vi "getLimitsByName.vi"(8 "error in (no error)":errorcluster, 10 "device_name":string, 11 "deviceDataBase in":refnum<class "deviceDataBase.lvclass">) -> (0 "error out":errorcluster, 2 "Limits":T1(array[cluster]), 3 "deviceDataBase out":refnum<class "deviceDataBase.lvclass">)   [LabVIEW 2011, in "Tools.lvlib" / "DatabaseHelpers.lvlib" / "deviceDataBase.lvclass"]
uses:
  deviceDataBase.lvclass
  deviceDataBase.lvclass/deviceDataBase.ctl
  Database Objects/device/device.lvclass
  Database Objects/device/AnalogDevice/AnalogDevice.lvclass
  Database Objects/DeviceArray/DeviceArray.lvclass
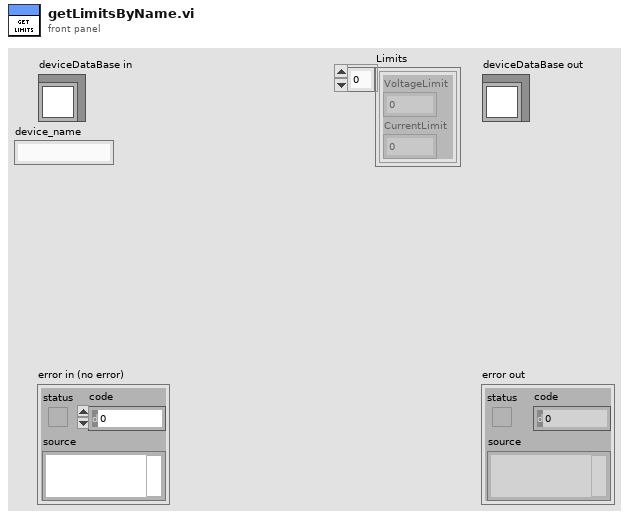
[diagram p1: front panel]
types:
  T1 = cluster{"VoltageLimit":dbl, "CurrentLimit":dbl}[]
  T2 = enum16{"digitalOutput", "digitalInput", "analogOutput", "analogInput", "rfOutput", "ethernetSupply"}
  T3 = cluster{"Range":cluster{"current":dbl, "voltage":dbl}, "triggering_inUse":cluster{"start_trigger":string, "clock":string}, "Limits":cluster{"VoltageLimit":dbl, "CurrentLimit":dbl}}[]
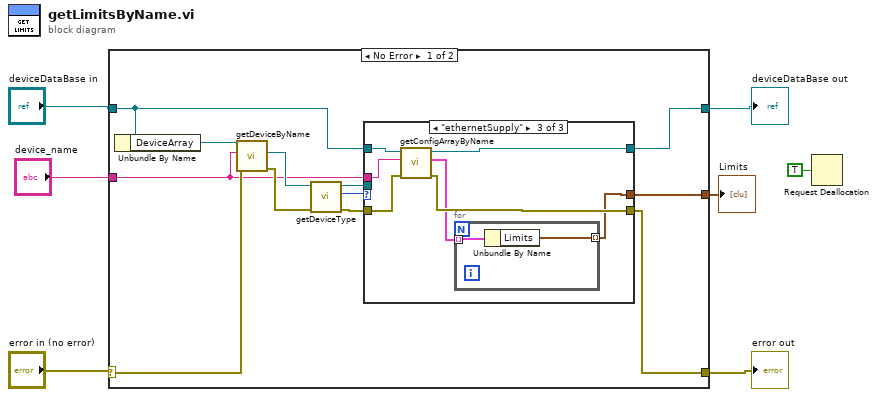
[diagram p0: block diagram]
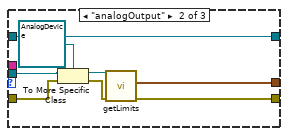
[diagram p3: hidden frame]
diagram:
  n1 = case shown="No Error" "error in (no error)" {
    selector: "error in (no error)" -> [w18 w40]
    tunnel: [w12 w40] -> w5
    tunnel: [w9 w39] -> w4
    tunnel: "deviceDataBase in" -> [w10 w39]
    tunnel: "device_name" -> [w8 _]
    tunnel: [w11 _] -> w2
    frame No Error {
      n2 = Unbundle By Name(w10) -> ("DeviceArray"=w19:refnum<class "DeviceArray.lvclass">)
      n3 = call "getDeviceByName.vi"("error in (no error)"=w18, "deviceName"=w8, "DeviceArray in"=w19) -> ("error out"=w16:errorcluster, "device.lvclass"=w17:refnum<class "device.lvclass">)  [unwired: 5 in, 2 out]
      n4 = call-dynamic "getDeviceType.vi"("error in (no error)"=w16, "device.lvclass in"=w17) -> ("error out"=w13:errorcluster, "type"=w15:T2, "device.lvclass out"=w14:refnum<class "device.lvclass">)  [unwired: 7 in]
      n5 = case shown="\"ethernetSupply\"" w15 {
        tunnel: w14 -> [_ w29 _]
        tunnel: w13 -> [w21 w25 w34]
        tunnel: [w21 w24 w33] -> w12
        tunnel: [_ w23 w30] -> w11
        tunnel: w10 -> [w20 w22 w36]
        tunnel: [w20 w22 w35] -> w9
        tunnel: w8 -> [_ _ w32]
        frame Default {
        }
        frame "analogOutput" {
          n6 = To More Specific Class(target class=refnum<class "AnalogDevice.lvclass"> refnum ("AnalogDevice in"), reference=w29, error in=w25) -> (specific class reference=w27:refnum<class "AnalogDevice.lvclass">, error out=w26:errorcluster)
          n7 = call "getLimits.vi"("error in (no error)"=w26, "AnalogDevice in"=w27) -> ("error out"=w24:errorcluster, "Limits"=w23:T1)  [unwired: 7 in, 1 out]
        }
        frame "ethernetSupply" {
          n8 = call "getConfigArrayByName.vi"("error in (no error)"=w34, "device_name"=w32, "deviceDataBase in"=w36) -> ("error out"=w33:errorcluster, "ConfigArray"=w31:T3, "deviceDataBase out"=w35:refnum<class "deviceDataBase.lvclass">)  [unwired: 6 in]
          n9 = for {
            tunnel: w31 -> [w38] mode=indexing
            tunnel: [w37] -> w30 mode=indexing
            n10 = Unbundle By Name(w38) -> ("Limits"=w37:cluster{"VoltageLimit":dbl, "CurrentLimit":dbl})
          }
        }
      }
    }
    frame Error {
    }
  }
  "error out" <- w5
  "deviceDataBase out" <- w4
  "Limits" <- w2
  n11 = Request Deallocation(TRUE ("flag")) -> ()
